vi "KE2260B Initialize.vi"(7 "Serial Configuration":T1={"Baud Rate"=9600, "Parity"=0, "Data Bits"=8, "Stop Bits"=10, "Flow Control"=0} {"Flow Control" items=["None", "XON/XOFF", "RTS/CTS", "XON/XOFF & RTS/CTS", "DTR/DSR", "XON/XOFF & DTR/DSR"]; "Stop Bits" items=["1.0"=10, "1.5"=15, "2.0"=20]; "Data Bits" items=["7"=7, "8"=8]; "Parity" items=["None", "Odd", "Even", "Mark", "Space"]; "Baud Rate" items=["300"=300, "600"=600, "1200"=1200, "2400"=2400, "4800"=4800, "9600"=9600, "19200"=19200]}, 8 "error in (no error)":errorcluster, 9 "Reset (True)":bool=TRUE, 10 "ID Query (True)":bool=TRUE, 11 "VISA resource name":refnum<visa-resource-name>) -> (0 "error out":errorcluster, 3 "VISA resource name out":refnum<visa-resource-name>)   [LabVIEW 2009, in "Keithley 2260B.lvlib"]
doc: "Establishes communication with the instrument and optionally performs an instrument identification query and/or an instrument reset. It also places the instrument in a default state needed for other instrument driver operations. Therefore, call this VI before calling other instrument driver VIs for this instrument. Generally, you need to call the Initialize VI only once at the beginning of an application."
uses:
  <instrlib>/Keithley 2260B/Keithley 2260B.lvlib
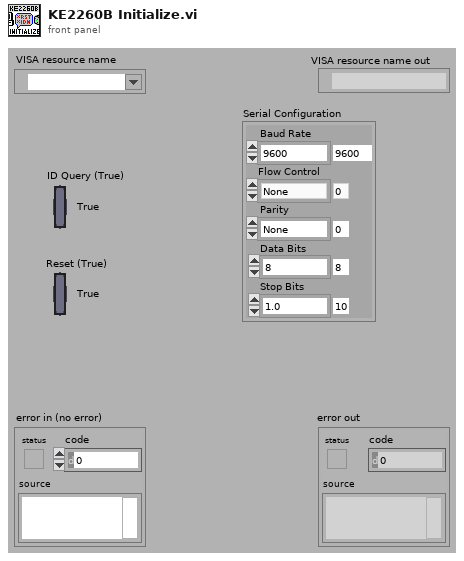
[diagram p1: front panel]
types:
  T1 = cluster{"Baud Rate":u32, "Parity":u16, "Data Bits":u16, "Stop Bits":u16, "Flow Control":u16}
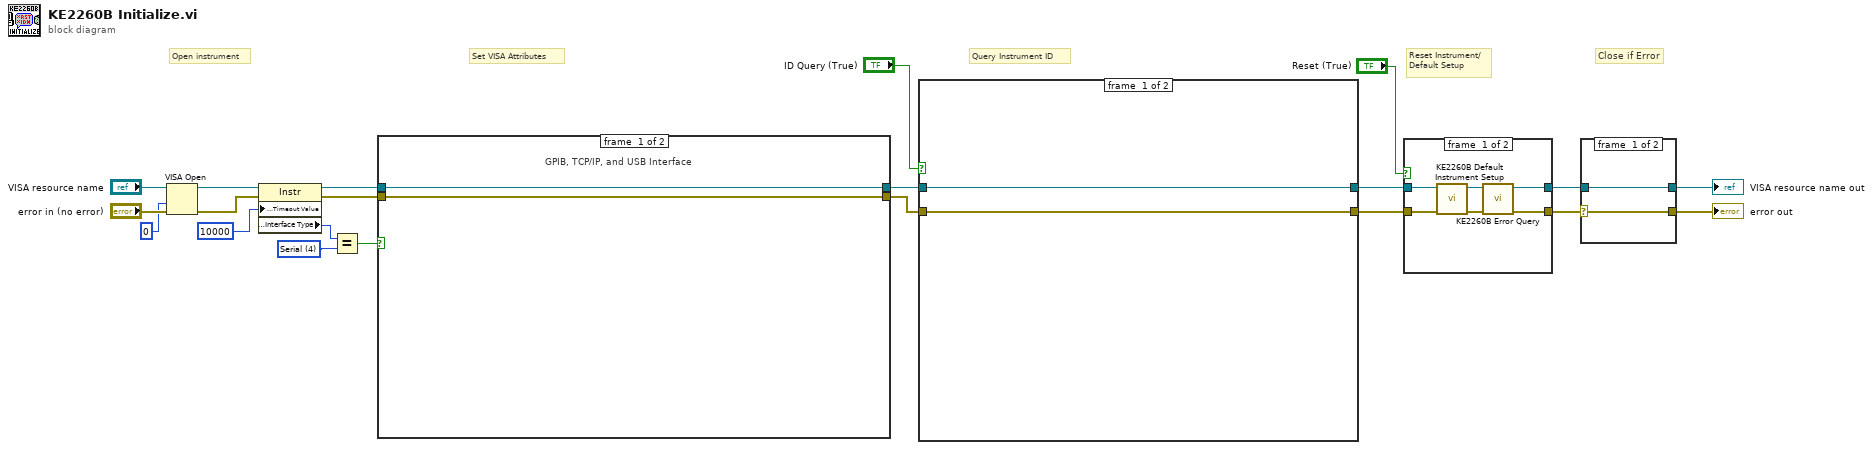
[diagram p0: block diagram]
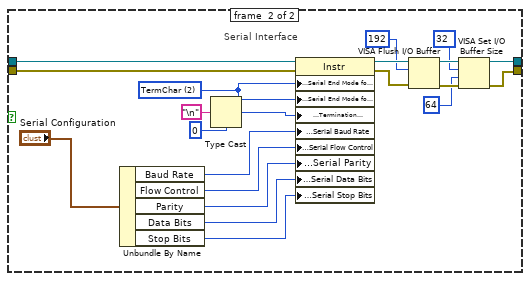
[diagram p2: hidden frame]
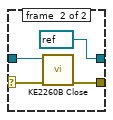
[diagram p3: hidden frame]
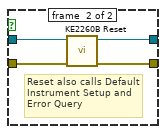
[diagram p4: hidden frame]
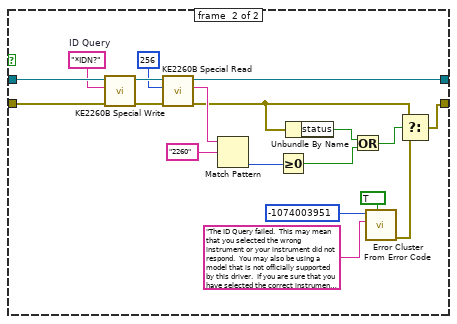
[diagram p5: hidden frame]
diagram:
  w8 = u16 4 items=["GPIB"=1, "VXI"=2, "GPIB-VXI"=3, "Serial"=4, "PXI"=5, "TCPIP"=6, "USB"=7] ("Interface Information:Interface Type")
  # "Set VISA Attributes"
  # "Close if Error"
  # "Query Instrument ID"
  # "Reset Instrument/\nDefault Setup"
  # "Open instrument"
  n1 = VISA Open(access mode=u32 0, error in (no error)="error in (no error)", VISA resource name="VISA resource name") -> (VISA resource name=w2:refnum<visa-resource-name>, error out=w1:errorcluster)  [unwired: 2 in]
  n2 = property class="Instr"(reference=w2, error in=w1, "General Settings:Timeout Value"=u32 10000) -> (reference out=w11:refnum<visa-resource-name>, error out=w10:errorcluster, "Interface Information:Interface Type"=w15:u16)
  n3 = Equal?(x=w15, y=w8) -> (x = y?=w9:bool)
  n4 = case shown="True" w9 {
    tunnel: [w22 w41] -> w13
    tunnel: [w23 w38] -> w12
    tunnel: w11 -> [w22 w43]
    tunnel: w10 -> [w23 w44]
    frame #0 {
      # "GPIB, TCP/IP, and USB Interface"
    }
    frame #1 {
      w32 = u16 2 items=["None", "LastBit", "TermChar"] ("Serial Settings:Serial End Mode for Reads")
      # "Serial Interface"
      n5 = Unbundle By Name("Serial Configuration") -> ("Baud Rate"=w30:u32, "Flow Control"=w26:u16, "Parity"=w28:u16, "Data Bits"=w29:u16, "Stop Bits"=w25:u16)
      n6 = Type Cast(type=u8 0, x="\n" ("Line Feed Constant")) -> (*(type *) &x=w31:u8)
      n7 = property class="Instr"(reference=w43, error in=w44, "Serial Settings:Serial End Mode for Reads"=w32, "Serial Settings:Serial End Mode for Writes"=w32, "Message Based Settings:Termination Character"=w31, "Serial Settings:Serial Baud Rate"=w30, "Serial Settings:Serial Flow Control"=w26, "Serial Settings:Serial Parity"=w28, "Serial Settings:Serial Data Bits"=w29, "Serial Settings:Serial Stop Bits"=w25) -> (reference out=w37:refnum<visa-resource-name>, error out=w40:errorcluster)
      n8 = VISA Flush I/O Buffer(VISA resource name=w37, mask (16)=u16 192, error in (no error)=w40) -> (VISA resource name out=w42:refnum<visa-resource-name>, error out=w39:errorcluster)
      n9 = VISA Set I/O Buffer Size(VISA resource name=w42, mask (16)=u16 32, size (4096)=u32 64 ("size (0)"), error in (no error)=w39) -> (VISA resource name out=w41:refnum<visa-resource-name>, error out=w38:errorcluster)
    }
  }
  n10 = case shown="True" "ID Query (True)" {
    tunnel: [w45 w65] -> w20
    tunnel: [w46 w62] -> w21
    tunnel: w13 -> [w46 w63]
    tunnel: w12 -> [w45 w64]
    frame #0 {
    }
    frame #1 {
      w56 = "*IDN?"  # ID Query
      n11 = call <instrlib>:"KE2260B Special Write.vi"("error in (no error)"=w64, "Write Buffer (\"\")"=w56, "VISA session"=w63) -> ("error out"=w59:errorcluster, "dup VISA session"=w60:refnum<visa-resource-name>)  [unwired: 6 in, 1 out]
      n12 = call <instrlib>:"KE2260B Special Read.vi"("error in (no error)"=w59, "byte count"=u32 256, "VISA session"=w60) -> ("error out"=w50:errorcluster, "read buffer"=w61:string, "dup VISA session"=w62:refnum<visa-resource-name>)  [unwired: 5 in, 1 out]
      n13 = Match Pattern(string=w61, regular expression="2260") -> (offset past match=w51:i32)  [unwired: 1 in, 3 out]
      n14 = Greater Or Equal To 0?(x=w51) -> (x >= 0?=w48:bool)
      n15 = Unbundle By Name(w50) -> ("status"=w49:bool)
      n16 = Or(x=w49, y=w48) -> (x .or. y?=w47:bool)
      n17 = call <vilib>:"Error Cluster From Error Code.vi"("show call chain? (False)"=TRUE, "error message (\"\")"="The ID Query failed.  This may mean that you selected the wrong instrument or your instrument did not respond.  You may also be using a model that is not officially supported by this driver.  If you are sure that you have selected the correct instrument and it is responding, try disabling the ID Query." ("Source (VI Name)"), "error code (0)"=-1074003951 ("Code")) -> ("error out"=w55:errorcluster)  [unwired: 6 in]
      n18 = Select(t=w50, s=w47, f=w55) -> (s? t:f=w65:errorcluster)
    }
  }
  n19 = case shown="True" "Reset (True)" {
    tunnel: w20 -> [w70 w72]
    tunnel: [w67 w75] -> w3
    tunnel: w21 -> [w71 w73]
    tunnel: [w68 w74] -> w4
    frame #0 {
      n20 = call <instrlib>:"KE2260B Default Instrument Setup.vi"("error in (no error)"=w70, "VISA resource name"=w71) -> ("error out"=w66:errorcluster, "VISA resource name out"=w69:refnum<visa-resource-name>)  [unwired: 8 in]
      n21 = call <instrlib>:"KE2260B Error Query.vi"("error in (no error)"=w66, "VISA resource name"=w69) -> ("error out"=w67:errorcluster, "VISA resource name out"=w68:refnum<visa-resource-name>)  [unwired: 6 in, 2 out]
    }
    frame #1 {
      # "Reset also calls Default Instrument Setup and Error Query"
      n22 = call <instrlib>:"KE2260B Reset.vi"("error in (no error)"=w72, "VISA resource name"=w73) -> ("error out"=w75:errorcluster, "VISA resource name out"=w74:refnum<visa-resource-name>)  [unwired: 8 in]
    }
  }
  n23 = case shown="Error" w3 {
    selector: w3 -> [w76 w79]
    tunnel: w4 -> [w77 w80]
    tunnel: [w77 refnum<visa-resource-name> refnum ("VISA resource name out")] -> w6
    tunnel: [w76 w81] -> w5
    frame #0 {
    }
    frame #1 {
      n24 = call <instrlib>:"KE2260B Close.vi"("error in (no error)"=w79, "VISA resource name"=w80) -> ("error out"=w81:errorcluster)  [unwired: 9 in]
    }
  }
  "VISA resource name out" <- w6
  "error out" <- w5
